vi "2020_day08.vi"() -> ()   [LabVIEW 2021]
panel:
  out "NOP to JMP: ACC":i32
  out "NOP to JMP: Reached End of Instruction List?":bool
  out "JMP to NOP: Reached End of Instruction List?":bool
  out "JMP to NOP: ACC":i32
  out "Last ACC (Task 1)":i32
  in  "Switch":bool caption="Ex. Data  vs.  User Data"
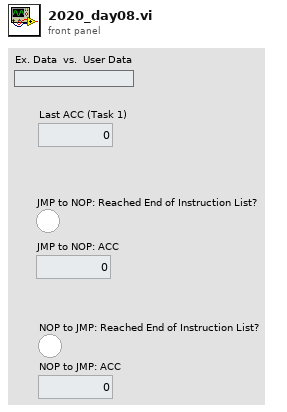
[diagram p1: front panel]
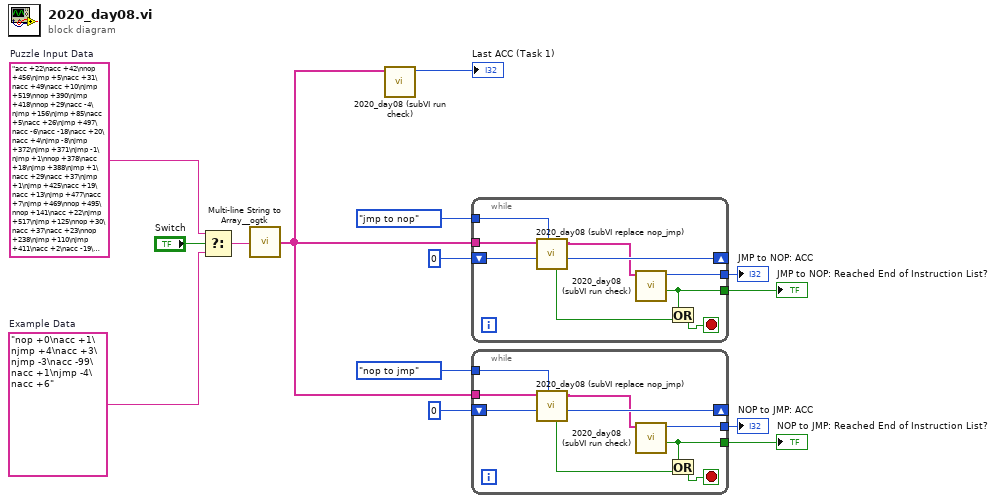
[diagram p0: block diagram]
diagram:
  w12 = "acc +22\nacc +42\nnop +456\njmp +5\nacc +31\nacc +49\nacc +10\njmp +519\nnop +390\njmp +418\nnop +29\nacc -4\njmp +156\njmp +85\nacc +5\nacc +26\njmp +497\nacc -6\nacc -18\nacc +20\nacc +4\njmp -8\njmp +372\njmp +371\njmp -1\njmp +1\nnop +378\nacc +18\njmp +388\njmp +1\nacc +29\nacc +37\njmp +1\njmp +425\nacc +19\nacc +13\njmp +477\nacc +7\njmp +469\nnop +495\nnop +141\nacc +22\njmp +517\njmp +125\nnop +30\nacc +37\nacc +23\nnop +238\njmp +110\njmp +411\nacc +2\nacc -19\nacc -19\njmp +296\nacc +0\nacc +14\nacc +20\njmp +75\nnop +88\nacc -16\nacc +40\nacc +27\njmp +131\nacc +33\nnop +252\nacc +5\nacc +0\njmp +101\nnop +219\nacc +50\nacc +40\njmp +49\nnop +74\njmp +327\nacc +47\njmp +206\nacc -15\njmp +449\nacc -17\nacc -13\nacc +46\njmp +417\njmp +160\nacc -7\nacc -11\nacc +16\nacc +14\njmp -37\nacc -12\nacc +15\nacc -14\nnop +110\njmp +1\nacc -4\nnop +287\nnop -82\njmp +30\njmp +490\nacc +34\njmp +305\nnop +90\njmp +1\nnop -4\nnop -95\njmp -46\nacc +26\nacc +13\nacc +47\njmp +350\nacc +11\njmp -102\nacc -2\njmp +489\nacc +28\nacc +24\nnop +486\njmp +485\nnop +170\njmp +66\njmp +411\nacc +30\nacc +48\nacc +48\njmp -6\nacc +11\njmp -51\njmp +1\njmp -10\nnop +411\nacc -17\nacc +32\njmp +9\njmp +398\nnop +82\njmp +6\nacc +45\nacc +34\njmp -44\nacc -13\njmp -122\nacc +25\nnop +286\nacc +5\njmp +144\nacc +0\njmp -122\nacc -11\nacc -6\njmp -123\nacc +16\nacc +1\njmp -58\nnop +242\nacc -11\njmp +257\nnop +231\nacc +46\njmp +301\nacc -6\nacc +20\nacc -7\njmp +365\nacc +32\nacc +0\njmp -66\njmp +110\nacc -18\njmp +118\nacc +33\nnop -125\nacc +49\nacc +36\njmp +188\nacc +9\nacc -11\njmp +100\nacc +35\njmp +55\nacc +38\nacc -1\njmp +312\njmp +157\nacc +17\njmp +177\nnop -126\nacc +30\nacc -3\njmp +211\nacc -3\njmp -164\njmp -112\nacc +50\njmp +268\nnop +290\nacc -8\nacc +35\njmp -44\nacc -6\nacc +11\nnop +327\njmp +155\nacc +10\nacc +35\nnop +233\njmp +330\nacc +31\nacc +8\njmp +124\nacc -5\njmp +300\nnop +171\nnop +4\nacc +19\nacc +41\njmp -156\nnop +179\nacc +12\njmp +160\njmp -92\nacc -11\nacc -10\njmp +95\nnop +94\nacc -8\njmp -199\nacc +16\nacc +30\nnop +73\nacc +36\njmp -53\njmp +1\njmp -6\nnop +369\nacc +29\nacc +47\njmp +32\nacc +35\njmp -61\nacc +41\njmp +352\nacc -1\njmp +75\nacc -10\nacc +28\nacc -15\njmp -187\nacc +6\njmp +1\nnop +112\njmp +273\nnop +186\nacc +11\nacc +40\njmp +128\nacc +17\nacc +23\nacc -8\nnop +277\njmp +42\nacc +11\nnop -237\nacc +36\nacc +32\njmp +287\nacc +16\nacc -19\njmp +115\nacc -6\nacc +16\nnop -2\nacc +23\njmp -160\nacc -10\nacc -10\njmp +26\nacc -7\njmp -95\nnop -160\nacc -2\nacc +44\njmp -236\njmp -198\njmp +1\nacc +1\njmp -9\njmp -95\njmp +273\nacc -19\njmp -46\nacc +12\nacc +2\njmp -145\nacc -14\nacc +3\nacc +3\njmp +250\nacc +4\nacc +40\njmp +1\njmp +17\nacc +6\nacc +47\njmp -77\nnop -192\nacc +11\njmp +296\nacc -14\njmp +64\nacc +35\njmp +134\nacc -8\nnop +228\nacc +24\nacc +15\njmp -64\njmp -241\nacc +19\nacc +22\nacc +49\nnop -193\njmp +219\nacc -1\nacc -11\nnop +211\nacc +0\njmp -106\nnop +101\njmp -222\nacc +20\nacc +45\njmp +70\nacc +19\nacc +21\njmp -23\nacc +8\nnop +92\nacc +47\njmp -144\nacc +0\nacc -1\njmp -81\nacc +23\njmp -274\nacc +14\nacc +26\nacc +9\njmp +79\nacc +22\njmp -331\nacc -10\njmp -311\nacc +16\nacc +30\nacc -8\njmp +176\nacc -19\nacc +43\njmp -222\nnop -116\njmp +18\nacc +26\nacc +23\nacc +6\njmp -162\nacc +34\njmp +95\nacc +27\nacc +40\nacc +9\njmp -77\njmp +137\nacc -13\nacc +21\nacc +17\nacc -5\njmp +91\njmp -95\nacc +18\nacc -1\njmp +70\njmp -355\nnop -166\nacc -19\nacc +16\njmp -146\njmp -135\njmp +57\nacc +45\njmp -62\nacc -14\njmp -382\nnop -172\nacc +45\njmp -77\nacc +13\njmp +65\nacc -4\njmp +112\njmp +107\njmp +26\njmp -326\nacc +25\njmp +1\njmp +179\nacc +33\nacc +2\njmp -222\nnop +36\nacc +25\nnop -244\njmp -376\njmp -203\nacc +26\nnop +109\nacc +38\njmp +135\nacc +7\nacc +40\nacc -18\njmp -113\nnop -294\nacc +0\nacc +40\nnop -265\njmp +81\njmp -99\njmp +32\nacc -17\nacc +25\nacc -12\nacc +26\njmp -125\nacc -3\nacc -7\nacc +25\njmp -410\nacc +47\nacc +36\njmp +35\nacc +2\nacc +18\nacc -3\njmp -38\nacc +29\nacc +49\njmp -299\nacc -4\nnop -422\njmp +50\nacc +11\nacc +2\nacc +49\njmp -233\nacc +12\nacc +43\nacc -19\nacc +11\njmp -264\njmp +124\njmp -361\nacc +35\njmp -118\nacc +23\nacc -16\nacc -14\njmp -22\njmp -135\njmp -309\nacc +6\njmp -44\nacc -12\nacc +0\njmp -23\nacc +29\nacc -8\nacc +18\nacc +35\njmp -111\nacc +22\nacc +23\nacc +0\nacc -8\njmp -55\nacc +14\njmp +1\nacc +44\nacc +17\njmp -272\nacc +39\nnop +37\nacc -19\njmp -323\nacc +24\nacc +28\nacc +29\nacc +37\njmp +110\njmp -386\nnop -352\nacc +23\nacc +38\njmp -369\nacc -5\nacc -14\njmp +83\njmp +17\njmp -151\njmp -118\njmp -104\njmp -341\nacc +32\nacc +43\njmp -52\nacc -4\nacc +42\nacc +5\njmp -116\nacc +13\njmp +1\nnop -361\nacc +41\njmp -386\njmp -241\nnop -449\nacc +46\njmp -176\nacc +6\njmp +60\njmp +1\njmp -3\njmp -62\nacc -14\nacc +17\njmp -340\nacc +31\nacc -13\nacc +7\njmp -54\njmp -80\nacc +14\nacc +49\nacc +34\njmp +24\nacc +11\njmp -158\nacc -13\njmp -261\nacc +33\nnop -171\njmp -106\nacc +0\nacc +9\nacc +16\nacc +34\njmp +18\nacc -2\nacc +47\nacc +39\njmp -232\nacc +23\nnop -229\nacc +30\nacc +32\njmp -147\nacc -8\njmp -460\njmp -498\nnop -218\nacc +31\nacc +44\nacc +30\njmp -105\nacc +8\nacc -19\nacc +45\nnop -49\njmp -140\nnop -43\nacc +42\njmp +1\nacc -14\njmp -42\njmp -389\nacc +39\nacc +26\nacc +38\njmp -77\nacc +48\njmp -83\nacc +5\njmp -81\nnop -242\nacc +35\nacc +0\nacc +19\njmp -430\nacc +11\nnop -226\nacc +13\nacc +23\njmp -575\nacc +44\nacc +50\nnop -303\njmp -112\njmp -305\nacc +23\nacc -11\nnop -376\nacc +50\njmp +1"  # Puzzle Input Data
  w13 = "nop +0\nacc +1\njmp +4\nacc +3\njmp -3\nacc -99\nacc +1\njmp -4\nacc +6"  # Example Data
  n1 = Select(t=w12, s="Switch", f=w13) -> (s? t:f=w11:string)
  n2 = call <userlib>:"Multi-line String to Array__ogtk.vi"("string"=w11) -> ("lines"=w1:string[])
  n3 = call "2020_day08 (subVI run check).vi"("lines"=w1) -> ("ACC"=→"Last ACC (Task 1)":i32)  [unwired: 9 in, 1 out]
  n4 = while {
    tunnel: w1 -> [w23]
    shift-right: [w21] -> _
    shift-left: 0 ("Start Line") -> [w22]
    tunnel: [w18] -> w6
    tunnel: [w19] -> w7
    tunnel: enum16{"jmp to nop", "nop to jmp"}."jmp to nop" ("Mode") -> [w15]
    stop <- w16 stop-if-true
    n5 = call "2020_day08 (subVI replace nop_jmp).vi"("Mode"=w15, "Start Line In"=w22, "Array In"=w23) -> ("Start Line Out"=w21:i32, "Array Out"=w20:string[], "End of Replacement Reached?"=w17:bool)  [unwired: 6 in]
    n6 = call "2020_day08 (subVI run check).vi"("lines"=w20) -> ("Reached End of Instruction List?"=w18:bool, "ACC"=w19:i32)  [unwired: 9 in]
    n7 = Or(x=w18, y=w17) -> (x .or. y?=w16:bool)
  }
  "JMP to NOP: ACC" <- w7
  "JMP to NOP: Reached End of Instruction List?" <- w6
  n8 = while {
    tunnel: w1 -> [w32]
    shift-right: [w30] -> _
    shift-left: 0 ("Start Line") -> [w31]
    tunnel: [w27] -> w5
    tunnel: [w28] -> w4
    tunnel: enum16{"jmp to nop", "nop to jmp"}."nop to jmp" ("Mode") -> [w24]
    stop <- w25 stop-if-true
    n9 = call "2020_day08 (subVI replace nop_jmp).vi"("Mode"=w24, "Start Line In"=w31, "Array In"=w32) -> ("Start Line Out"=w30:i32, "Array Out"=w29:string[], "End of Replacement Reached?"=w26:bool)  [unwired: 6 in]
    n10 = call "2020_day08 (subVI run check).vi"("lines"=w29) -> ("Reached End of Instruction List?"=w27:bool, "ACC"=w28:i32)  [unwired: 9 in]
    n11 = Or(x=w27, y=w26) -> (x .or. y?=w25:bool)
  }
  "NOP to JMP: ACC" <- w4
  "NOP to JMP: Reached End of Instruction List?" <- w5
